vi "Compile Routing and Faulting Configuration.vi"(6 "Get Channel Data Refnum":refnum<vi>, 8 "error in (no error)":errorcluster, 11 "Device Ref in":T1 format="%.0x") -> (0 "error out":errorcluster, 2 "RaF Configuration":T2, 3 "Device Ref out":T1 format="%.0x")   [LabVIEW 2017, in "Routing and Faulting System Explorer.lvlib"]
uses:
  Routing and Faulting System Explorer.lvlib
  Shared/Routing and Faulting Configuration.ctl
  Shared/Routing Channel Configuration.ctl
  Shared/Value-Connections Map.ctl
  Shared/Connection.ctl
  Shared/Alias Mapping.ctl
  <vilib>/NI Veristand/Custom Device API/Custom Device Item Ref.ctl
  Shared/Routing and Faulting Shared.lvlib
  <vilib>/NI VeriStand/Custom Device API/Custom Device API.lvlib
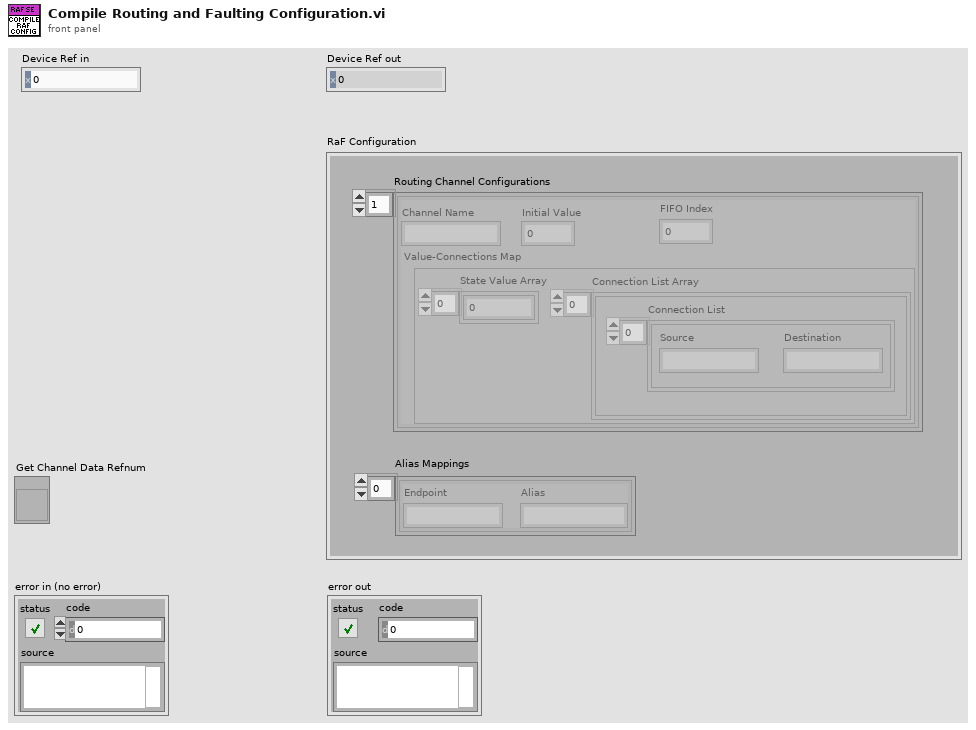
[diagram p1: front panel]
types:
  T1 = typedef "Custom Device API.lvlib/Custom Device Item Ref.ctl" = u64
  T2 = typedef "Routing and Faulting Shared.lvlib/Routing and Faulting Configuration.ctl" = cluster{"Routing Channel Configurations":T3[], "Alias Mappings":T6[]}
  T3 = typedef "Routing and Faulting Shared.lvlib/Routing Channel Configuration.ctl" = cluster{"Channel Name":string, "Initial Value":dbl, "FIFO Index":i32, "Value-Connections Map":T4}
  T4 = typedef "Routing and Faulting Shared.lvlib/Value-Connections Map.ctl" = cluster{"State Value Array":i32[], "Connection List Array":cluster{"Connection List":T5[]}[]}
  T5 = typedef "Routing and Faulting Shared.lvlib/Connection.ctl" = cluster{"Source":string, "Destination":string}
  T6 = typedef "Routing and Faulting Shared.lvlib/Alias Mapping.ctl" = cluster{"Endpoint":string, "Alias":string}
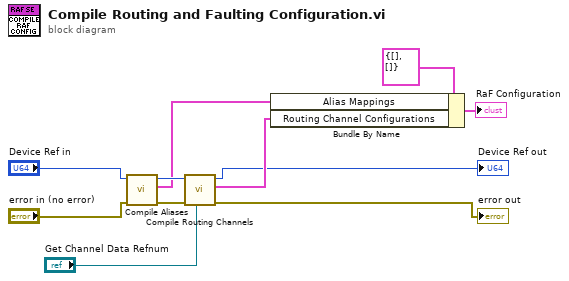
[diagram p0: block diagram]
diagram:
  n1 = call "Compile Aliases.vi"("error in (no error)"="error in (no error)", "Device Ref in"="Device Ref in") -> ("error out"=w6:errorcluster, "Alias Mappings"=w2:T6[], "Device Ref out"=w7:T1)  [unwired: 7 in]
  n2 = call "Compile Routing Channels.vi"("Get Channel Data Refnum"="Get Channel Data Refnum", "error in (no error)"=w6, "Device Ref in"=w7) -> ("error out"=→"error out":errorcluster, "Routing Channels Configuration"=w5:T3[], "Device Ref out"=→"Device Ref out":T1)  [unwired: 6 in]
  n3 = Bundle By Name(cluster=T2 {"Routing Channel Configurations"=[], "Alias Mappings"=[]} ("Routing and Faulting Configuration"), "Alias Mappings"=w2, "Routing Channel Configurations"=w5) -> (→"RaF Configuration":T2)
